vi "SysDef.Import.vi"(8 "error in (no error)":errorcluster, 11 "Path in":path) -> (0 "error out":errorcluster, 3 "Configuration":T1 {"DID Outputs"."Frames"."Signals"."Byte Order" items=["Little Endian", "Big Endian"]; "DID Outputs"."Frames"."Signals"."Data Type" items=["Signed", "Unsigned", "IEEE Float"]; "Memory Inputs"."Frames"."Signals"."Byte Order" items=["Little Endian", "Big Endian"]; "Memory Inputs"."Frames"."Signals"."Data Type" items=["Signed", "Unsigned", "IEEE Float"]; "Memory Outputs"."Frames"."Signals"."Byte Order" items=["Little Endian", "Big Endian"]; "Memory Outputs"."Frames"."Signals"."Data Type" items=["Signed", "Unsigned", "IEEE Float"]; "Routines"."Routine Array"."Stop Parameters"."Response"."Byte Order" items=["Little Endian", "Big Endian"]; "Routines"."Routine Array"."Stop Parameters"."Response"."Data Type" items=["Signed", "Unsigned", "IEEE Float"]; "Routines"."Routine Array"."Stop Parameters"."Cmd"."Byte Order" items=["Little Endian", "Big Endian"]; "Routines"."Routine Array"."Stop Parameters"."Cmd"."Data Type" items=["Signed", "Unsigned", "IEEE Float"]; "Routines"."Routine Array"."Request Parameters"."Response"."Byte Order" items=["Little Endian", "Big Endian"]; "Routines"."Routine Array"."Request Parameters"."Response"."Data Type" items=["Signed", "Unsigned", "IEEE Float"]; "Routines"."Routine Array"."Request Parameters"."Cmd"."Byte Order" items=["Little Endian", "Big Endian"]; "Routines"."Routine Array"."Request Parameters"."Cmd"."Data Type" items=["Signed", "Unsigned", "IEEE Float"]; "Routines"."Routine Array"."Start Parameters"."Response"."Byte Order" items=["Little Endian", "Big Endian"]; "Routines"."Routine Array"."Start Parameters"."Response"."Data Type" items=["Signed", "Unsigned", "IEEE Float"]; "Routines"."Routine Array"."Start Parameters"."Cmd"."Byte Order" items=["Little Endian", "Big Endian"]; "Routines"."Routine Array"."Start Parameters"."Cmd"."Data Type" items=["Signed", "Unsigned", "IEEE Float"]; "IO Controls"."IO Control Array"."Signals"."Response"."Byte Order" items=["Little Endian", "Big Endian"]; "IO Controls"."IO Control Array"."Signals"."Response"."Data Type" items=["Signed", "Unsigned", "IEEE Float"]; "IO Controls"."IO Control Array"."Signals"."Cmd"."Byte Order" items=["Little Endian", "Big Endian"]; "IO Controls"."IO Control Array"."Signals"."Cmd"."Data Type" items=["Signed", "Unsigned", "IEEE Float"]; "DTC"."DTC Control"."Signals"."Byte Order" items=["Little Endian", "Big Endian"]; "DTC"."DTC Control"."Signals"."Data Type" items=["Signed", "Unsigned", "IEEE Float"]; "Diagnostics Basic Configuraiton"."Fill Byte" format="%.0x"; "Diagnostics Basic Configuraiton"."VW TP Channel ID" format="%.0x"; "Diagnostics Basic Configuraiton"."Receive UUDT ID" format="%.0x"; "Diagnostics Basic Configuraiton"."Receive Extension" format="%.0x"; "Diagnostics Basic Configuraiton"."Transmit Extension" format="%.0x"; "Diagnostics Basic Configuraiton"."Receive ID" format="%.0x"; "Diagnostics Basic Configuraiton"."Transmit ID" format="%.0x"; "DID Inputs"."Frames"."Signals"."Byte Order" items=["Little Endian", "Big Endian"]; "DID Inputs"."Frames"."Signals"."Data Type" items=["Signed", "Unsigned", "IEEE Float"]; "PID Inputs"."Frames"."Signals"."Byte Order" items=["Little Endian", "Big Endian"]; "PID Inputs"."Frames"."Signals"."Data Type" items=["Signed", "Unsigned", "IEEE Float"]; "PID Outputs"."Frames"."Signals"."Byte Order" items=["Little Endian", "Big Endian"]; "PID Outputs"."Frames"."Signals"."Data Type" items=["Signed", "Unsigned", "IEEE Float"]})   [LabVIEW 2015, in "Diagnostics Addon System Explorer.lvlib"]
uses:
  Diagnostics Addon System Explorer.lvlib
  Types/SysDef.Export.ctl
  Shared/Types/CAN.ctl
  Shared/Types/CAN.Interface.ctl
  Shared/Types/Protocol.ctl
  Shared/Types/Transport.ctl
  Shared/Types/Security.ctl
  Types/Frames.Export.ctl
  Types/Frame.Export.ctl
  Shared/Types/Signal.ctl
  Types/DPIDs.Export.ctl
  Types/DPID.Export.ctl
  Shared/Types/DPID.ctl
  Shared/Types/DPID.Rate.ctl
  Types/DTC.Export.ctl
  Shared/Types/DTCDescriptor.ctl
  Types/DTCControl.Export.ctl
  Shared/Types/986x.ctl
  Types/Command.Export.ctl
  Types/Status.Export.ctl
  Types/IOControls.Export.ctl
  Types/IO.Export.ctl
  Types/CmdResp.Export.ctl
  Types/Routines.Export.ctl
  Types/Routine.Export.ctl
  Types/UserDefined.Export.ctl
  Types/UserDefined.Group.Export.ctl
  Types/UserDefined.Group.Message.Export.ctl
  <vilib>/NI/GXML/_subVIs/GXML SearchParser/Search Parser.vi
  <vilib>/NI/GXML/GXML.lvlib
  Shared/Diagnostics Addon Shared.lvlib
types:
  T1 = typedef "Diagnostics Addon System Explorer.lvlib/SysDef.Export.ctl" = cluster{"Name":string, "Description":string, "Diagnostics Basic Configuraiton":T2, "DID Outputs":T7, "DID Inputs":T7, "PID Outputs":T7, "PID Inputs":T7, "DPIDs":T10, "DTC":T14, "NI 986x Support":T17, "Commands":T18, "Status":T19, "IO Controls":T20, "Routines":T23, "Memory Outputs":T7, "Memory Inputs":T7, "User Defined":T25}
  T2 = typedef "Diagnostics Addon Shared.lvlib/CAN.ctl" = cluster{"CAN Interface":T3, "Baud Rate":u32, "Diagnostic Protocol":T4, "Transport Protocol":T5, "Transmit ID":u32, "Receive ID":u32, "Transmit Extension":u8, "Receive Extension":u8, "Receive UUDT ID":u32, "Enable Stream":bool, "VW TP Channel ID":u32, "Security":T6, "Fill Frame":bool, "Fill Byte":u8, "Termination":bool}
  T3 = typedef "Diagnostics Addon Shared.lvlib/CAN.Interface.ctl" = string
  T4 = typedef "Diagnostics Addon Shared.lvlib/Protocol.ctl" = enum16{"GMLAN", "KWP-2000", "UDS", "User-Defined"}
  T5 = typedef "Diagnostics Addon Shared.lvlib/Transport.ctl" = enum16{"ISO TP - Normal Mode", "ISO TP - Mixed Mode", "VW TP 2.0", "Diagnostics on IP"}
  T6 = typedef "Diagnostics Addon Shared.lvlib/Security.ctl" = cluster{"Source DLL Path":path, "Security Level":u8, "Target DLL Path":path}
  T7 = typedef "Diagnostics Addon System Explorer.lvlib/Frames.Export.ctl" = cluster{"Description":string, "Frames":T8[]}
  T8 = typedef "Diagnostics Addon System Explorer.lvlib/Frame.Export.ctl" = cluster{"Name":string, "Description":string, "ID":u32, "Signals":T9[]}
  T9 = typedef "Diagnostics Addon Shared.lvlib/Signal.ctl" = cluster{"Start Bit":u32, "Length":u32, "Scaling Factor":dbl, "Scaling Offset":dbl, "Minimum":dbl, "Maximum":dbl, "Data Type":u32, "Byte Order":u32, "Default Value":dbl, "Name":string, "Units":string, "Description":string}
  T10 = typedef "Diagnostics Addon System Explorer.lvlib/DPIDs.Export.ctl" = cluster{"Description":string, "DPIDs":T11[]}
  T11 = typedef "Diagnostics Addon System Explorer.lvlib/DPID.Export.ctl" = cluster{"Name":string, "Description":string, "DPID":T12}
  T12 = typedef "Diagnostics Addon Shared.lvlib/DPID.ctl" = cluster{"DPID ID":u8, "Speed":T13, "PIDs":u16[]}
  T13 = typedef "Diagnostics Addon Shared.lvlib/DPID.Rate.ctl" = enum16{"Slow", "Medium", "Fast"}
  T14 = typedef "Diagnostics Addon System Explorer.lvlib/DTC.Export.ctl" = cluster{"Description":string, "DTC descriptor":T15, "DTC Control":T16, "Created DTCs":u32}
  T15 = typedef "Diagnostics Addon Shared.lvlib/DTCDescriptor.ctl" = cluster{"DTC Byte Length":i32, "Status Byte Length":i32, "Add Data Byte Length":i32, "Byte Order":enum16{"Motorola", "Intel"}}
  T16 = typedef "Diagnostics Addon System Explorer.lvlib/DTCControl.Export.ctl" = cluster{"Description":string, "Signals":T9[]}
  T17 = typedef "Diagnostics Addon Shared.lvlib/986x.ctl" = cluster{"Enable":bool, "RIO Device":string, "Bitfile":path}
  T18 = typedef "Diagnostics Addon System Explorer.lvlib/Command.Export.ctl" = cluster{"Description":string}
  T19 = typedef "Diagnostics Addon System Explorer.lvlib/Status.Export.ctl" = cluster{"Description":string}
  T20 = typedef "Diagnostics Addon System Explorer.lvlib/IOControls.Export.ctl" = cluster{"Description":string, "IO Control Array":T21[]}
  T21 = typedef "Diagnostics Addon System Explorer.lvlib/IO.Export.ctl" = cluster{"Name":string, "Description":string, "ID":u16, "Signals":T22}
  T22 = typedef "Diagnostics Addon System Explorer.lvlib/CmdResp.Export.ctl" = cluster{"Cmd":T9[], "Response":T9[]}
  T23 = typedef "Diagnostics Addon System Explorer.lvlib/Routines.Export.ctl" = cluster{"Description":string, "Routine Array":T24[]}
  T24 = typedef "Diagnostics Addon System Explorer.lvlib/Routine.Export.ctl" = cluster{"Name":string, "Description":string, "ID":u16, "Start Parameters":T22, "Request Parameters":T22, "Stop Parameters":T22}
  T25 = typedef "Diagnostics Addon System Explorer.lvlib/UserDefined.Export.ctl" = cluster{"Description":string, "Groups":T26[]}
  T26 = typedef "Diagnostics Addon System Explorer.lvlib/UserDefined.Group.Export.ctl" = cluster{"Name":string, "Description":string, "Messages":T27[]}
  T27 = typedef "Diagnostics Addon System Explorer.lvlib/UserDefined.Group.Message.Export.ctl" = cluster{"Name":string, "Description":string, "Signals":T22}
  T28 = cluster{"Name":string, "Description":string, "Diagnostics Basic Configuraiton":cluster{"Database File":path, "CAN Interface":enum16{"CAN0", "CAN1", "CAN2", "CAN3", "CAN4", "CAN5", "CAN6", "CAN7", "CAN8", "CAN9", "CAN10", "CAN11", "CAN12", "CAN13", "CAN14", "CAN15", "CAN16", "CAN17", "CAN18", "CAN19", "CAN20", "CAN21", "CAN22", "CAN23", "CAN24", "CAN25", "CAN26", "CAN27", "CAN28", "CAN29", "CAN30", "CAN31", "CAN32", "CAN33", "CAN34", "CAN35", "CAN36", "CAN37", "CAN38", "CAN39", "CAN40", "CAN41", "CAN42", "CAN43", "CAN44", "CAN45", "CAN46", "CAN47", "CAN48", "CAN49", "CAN50", "CAN51", "CAN52", "CAN53", "CAN54", "CAN55", "CAN56", "CAN57", "CAN58", "CAN59", "CAN60", "CAN61", "CAN62", "CAN63", "CAN 256 (Virtual)", "CAN 257 (Virtual)"}, "Baud Rate":u32, "Diagnostic Protocol":enum16{"GMLAN", "KWP-2000", "UDS"}, "Transport Protocol":enum16{"ISO TP - Normal Mode", "ISO TP - Mixed Mode", "VW TP 2.0", "Diagnostics on IP"}, "Transmit ID":u32, "Receive ID":u32, "Transmit Extension":u8, "Receive Extension":u8, "Receive UUDT ID":u32, "Enable Stream":bool, "VW TP Channel ID":u32}, "DIDs":cluster{"Description":string, "DIDPID Array":cluster{"Name":string, "Description":string, "ID":u16, "Signals":cluster{"Name":string, "Start Bit":u8, "Length":u8, "Scaling Factor":dbl, "Scaling Offset":dbl, "Minimum":dbl, "Maximum":dbl, "Data Type":u32, "Byte Order":u32, "Default Value":dbl, "Units":string, "Description":string}[]}[]}, "Input PIDs":cluster{"Description":string, "DIDPID Array":cluster{"Name":string, "Description":string, "ID":u16, "Signals":cluster{"Name":string, "Start Bit":u8, "Length":u8, "Scaling Factor":dbl, "Scaling Offset":dbl, "Minimum":dbl, "Maximum":dbl, "Data Type":u32, "Byte Order":u32, "Default Value":dbl, "Units":string, "Description":string}[]}[]}, "Output PIDs":cluster{"Description":string, "DIDPID Array":cluster{"Name":string, "Description":string, "ID":u16, "Signals":cluster{"Name":string, "Start Bit":u8, "Length":u8, "Scaling Factor":dbl, "Scaling Offset":dbl, "Minimum":dbl, "Maximum":dbl, "Data Type":u32, "Byte Order":u32, "Default Value":dbl, "Units":string, "Description":string}[]}[]}, "DPIDs":cluster{"Description":string, "DPIDs":cluster{"Name":string, "Description":string, "DPID":cluster{"DPID ID":u8, "Speed":enum16{"Slow", "Medium", "Fast"}, "PIDs":u16[]}}[]}, "DTC":cluster{"Description":string, "DTC descriptor":cluster{"DTC Byte Length":i32, "Status Byte Length":i32, "Add Data Byte Length":i32, "Byte Order":enum16{"Motorola", "Intel"}}}, "NI 986x Support":cluster{"Enable 986x":bool, "RIO Device":u16, "Bitfile":path}, "Commands":cluster{"Description":string}, "Status":cluster{"Description":string}}
  T29 = cluster{"Description":string, "DPIDs":cluster{"Name":string, "Description":string, "DPID":cluster{"DPID ID":u8, "Speed":enum16{"Slow", "Medium", "Fast"}, "PIDs":u16[]}}[]}
  T30 = cluster{"DTC Byte Length":i32, "Status Byte Length":i32, "Add Data Byte Length":i32, "Byte Order":enum16{"Motorola", "Intel"}}
  T31 = enum16{"CAN0", "CAN1", "CAN2", "CAN3", "CAN4", "CAN5", "CAN6", "CAN7", "CAN8", "CAN9", "CAN10", "CAN11", "CAN12", "CAN13", "CAN14", "CAN15", "CAN16", "CAN17", "CAN18", "CAN19", "CAN20", "CAN21", "CAN22", "CAN23", "CAN24", "CAN25", "CAN26", "CAN27", "CAN28", "CAN29", "CAN30", "CAN31", "CAN32", "CAN33", "CAN34", "CAN35", "CAN36", "CAN37", "CAN38", "CAN39", "CAN40", "CAN41", "CAN42", "CAN43", "CAN44", "CAN45", "CAN46", "CAN47", "CAN48", "CAN49", "CAN50", "CAN51", "CAN52", "CAN53", "CAN54", "CAN55", "CAN56", "CAN57", "CAN58", "CAN59", "CAN60", "CAN61", "CAN62", "CAN63", "CAN 256 (Virtual)", "CAN 257 (Virtual)"}
  T32 = enum16{"ISO TP - Normal Mode", "ISO TP - Mixed Mode", "VW TP 2.0", "Diagnostics on IP"}
  T33 = cluster{"Name":string, "Description":string, "ID":u16, "Signals":cluster{"Name":string, "Start Bit":u8, "Length":u8, "Scaling Factor":dbl, "Scaling Offset":dbl, "Minimum":dbl, "Maximum":dbl, "Data Type":u32, "Byte Order":u32, "Default Value":dbl, "Units":string, "Description":string}[]}[]
  T34 = cluster{"Name":string, "Description":string, "Diagnostics Basic Configuraiton":cluster{"Database File":path, "CAN Interface":enum16{"CAN0", "CAN1", "CAN2", "CAN3", "CAN4", "CAN5", "CAN6", "CAN7", "CAN8", "CAN9", "CAN10", "CAN11", "CAN12", "CAN13", "CAN14", "CAN15", "CAN16", "CAN17", "CAN18", "CAN19", "CAN20", "CAN21", "CAN22", "CAN23", "CAN24", "CAN25", "CAN26", "CAN27", "CAN28", "CAN29", "CAN30", "CAN31", "CAN32", "CAN33", "CAN34", "CAN35", "CAN36", "CAN37", "CAN38", "CAN39", "CAN40", "CAN41", "CAN42", "CAN43", "CAN44", "CAN45", "CAN46", "CAN47", "CAN48", "CAN49", "CAN50", "CAN51", "CAN52", "CAN53", "CAN54", "CAN55", "CAN56", "CAN57", "CAN58", "CAN59", "CAN60", "CAN61", "CAN62", "CAN63", "CAN 256 (Virtual)", "CAN 257 (Virtual)"}, "Baud Rate":u32, "Diagnostic Protocol":enum16{"GMLAN", "KWP-2000", "UDS"}, "Transport Protocol":enum16{"ISO TP - Normal Mode", "ISO TP - Mixed Mode", "VW TP 2.0", "Diagnostics on IP"}, "Transmit ID":u32, "Receive ID":u32, "Transmit Extension":u8, "Receive Extension":u8, "Receive UUDT ID":u32, "Enable Stream":bool, "VW TP Channel ID":u32}, "DIDs":cluster{"Description":string, "DIDPID Array":cluster{"Name":string, "Description":string, "ID":u16, "Signals":cluster{"Start Bit":u8, "Length":u8, "Scaling Factor":dbl, "Scaling Offset":dbl, "Minimum":dbl, "Maximum":dbl, "Data Type":u32, "Byte Order":u32, "Default Value":dbl, "Name":string, "Units":string, "Description":string}[]}[]}, "Input PIDs":cluster{"Description":string, "DIDPID Array":cluster{"Name":string, "Description":string, "ID":u16, "Signals":cluster{"Start Bit":u8, "Length":u8, "Scaling Factor":dbl, "Scaling Offset":dbl, "Minimum":dbl, "Maximum":dbl, "Data Type":u32, "Byte Order":u32, "Default Value":dbl, "Name":string, "Units":string, "Description":string}[]}[]}, "Output PIDs":cluster{"Description":string, "DIDPID Array":cluster{"Name":string, "Description":string, "ID":u16, "Signals":cluster{"Start Bit":u8, "Length":u8, "Scaling Factor":dbl, "Scaling Offset":dbl, "Minimum":dbl, "Maximum":dbl, "Data Type":u32, "Byte Order":u32, "Default Value":dbl, "Name":string, "Units":string, "Description":string}[]}[]}, "DPIDs":cluster{"Description":string, "DPIDs":cluster{"Name":string, "Description":string, "DPID":cluster{"DPID ID":u8, "Speed":enum16{"Slow", "Medium", "Fast"}, "PIDs":u16[]}}[]}, "DTC":cluster{"Description":string, "DTC descriptor":cluster{"DTC Byte Length":i32, "Status Byte Length":i32, "Add Data Byte Length":i32, "Byte Order":enum16{"Motorola", "Intel"}}}, "NI 986x Support":cluster{"Enable 986x":bool, "RIO Device":u16, "Bitfile":path}, "Commands":cluster{"Description":string}, "Status":cluster{"Description":string}}
  T35 = cluster{"Name":string, "Description":string, "ID":u16, "Signals":cluster{"Start Bit":u8, "Length":u8, "Scaling Factor":dbl, "Scaling Offset":dbl, "Minimum":dbl, "Maximum":dbl, "Data Type":u32, "Byte Order":u32, "Default Value":dbl, "Name":string, "Units":string, "Description":string}[]}[]
  T36 = cluster{"Name":string, "Description":string, "Diagnostics Basic Configuraiton":cluster{"CAN Interface":enum16{"CAN0", "CAN1", "CAN2", "CAN3", "CAN4", "CAN5", "CAN6", "CAN7", "CAN8", "CAN9", "CAN10", "CAN11", "CAN12", "CAN13", "CAN14", "CAN15", "CAN16", "CAN17", "CAN18", "CAN19", "CAN20", "CAN21", "CAN22", "CAN23", "CAN24", "CAN25", "CAN26", "CAN27", "CAN28", "CAN29", "CAN30", "CAN31", "CAN32", "CAN33", "CAN34", "CAN35", "CAN36", "CAN37", "CAN38", "CAN39", "CAN40", "CAN41", "CAN42", "CAN43", "CAN44", "CAN45", "CAN46", "CAN47", "CAN48", "CAN49", "CAN50", "CAN51", "CAN52", "CAN53", "CAN54", "CAN55", "CAN56", "CAN57", "CAN58", "CAN59", "CAN60", "CAN61", "CAN62", "CAN63", "CAN 256 (Virtual)", "CAN 257 (Virtual)"}, "Baud Rate":u32, "Diagnostic Protocol":enum16{"GMLAN", "KWP-2000", "UDS"}, "Transport Protocol":enum16{"ISO TP - Normal Mode", "ISO TP - Mixed Mode", "VW TP 2.0", "Diagnostics on IP"}, "Transmit ID":u32, "Receive ID":u32, "Transmit Extension":u8, "Receive Extension":u8, "Receive UUDT ID":u32, "Enable Stream":bool, "VW TP Channel ID":u32, "Security":cluster{"Source DLL Path":path, "Security Level":u8, "Target DLL Path":path}, "Fill Frame":bool, "Fill Byte":u8, "Termination":bool}, "DID Outputs":cluster{"Description":string, "Frames":cluster{"Name":string, "Description":string, "ID":u32, "Signals":cluster{"Start Bit":u8, "Length":u8, "Scaling Factor":dbl, "Scaling Offset":dbl, "Minimum":dbl, "Maximum":dbl, "Data Type":u32, "Byte Order":u32, "Default Value":dbl, "Name":string, "Units":string, "Description":string}[]}[]}, "DID Inputs":cluster{"Description":string, "Frames":cluster{"Name":string, "Description":string, "ID":u32, "Signals":cluster{"Start Bit":u8, "Length":u8, "Scaling Factor":dbl, "Scaling Offset":dbl, "Minimum":dbl, "Maximum":dbl, "Data Type":u32, "Byte Order":u32, "Default Value":dbl, "Name":string, "Units":string, "Description":string}[]}[]}, "PID Outputs":cluster{"Description":string, "Frames":cluster{"Name":string, "Description":string, "ID":u32, "Signals":cluster{"Start Bit":u8, "Length":u8, "Scaling Factor":dbl, "Scaling Offset":dbl, "Minimum":dbl, "Maximum":dbl, "Data Type":u32, "Byte Order":u32, "Default Value":dbl, "Name":string, "Units":string, "Description":string}[]}[]}, "PID Inputs":cluster{"Description":string, "Frames":cluster{"Name":string, "Description":string, "ID":u32, "Signals":cluster{"Start Bit":u8, "Length":u8, "Scaling Factor":dbl, "Scaling Offset":dbl, "Minimum":dbl, "Maximum":dbl, "Data Type":u32, "Byte Order":u32, "Default Value":dbl, "Name":string, "Units":string, "Description":string}[]}[]}, "DPIDs":cluster{"Description":string, "DPIDs":cluster{"Name":string, "Description":string, "DPID":cluster{"DPID ID":u8, "Speed":enum16{"Slow", "Medium", "Fast"}, "PIDs":u16[]}}[]}, "DTC":cluster{"Description":string, "DTC descriptor":cluster{"DTC Byte Length":i32, "Status Byte Length":i32, "Add Data Byte Length":i32, "Byte Order":enum16{"Motorola", "Intel"}}, "DTC Control":cluster{"Description":string, "Signals":cluster{"Start Bit":u8, "Length":u8, "Scaling Factor":dbl, "Scaling Offset":dbl, "Minimum":dbl, "Maximum":dbl, "Data Type":u32, "Byte Order":u32, "Default Value":dbl, "Name":string, "Units":string, "Description":string}[]}}, "NI 986x Support":cluster{"Enable":bool, "RIO Device":u16, "Bitfile":path}, "Commands":cluster{"Description":string}, "Status":cluster{"Description":string}, "IO Controls":cluster{"Description":string, "IO Control Array":cluster{"Name":string, "Description":string, "ID":u16, "Signals":cluster{"Cmd":cluster{"Start Bit":u8, "Length":u8, "Scaling Factor":dbl, "Scaling Offset":dbl, "Minimum":dbl, "Maximum":dbl, "Data Type":u32, "Byte Order":u32, "Default Value":dbl, "Name":string, "Units":string, "Description":string}[], "Response":cluster{"Start Bit":u8, "Length":u8, "Scaling Factor":dbl, "Scaling Offset":dbl, "Minimum":dbl, "Maximum":dbl, "Data Type":u32, "Byte Order":u32, "Default Value":dbl, "Name":string, "Units":string, "Description":string}[]}}[]}, "Routines":cluster{"Description":string, "Routine Array":cluster{"Name":string, "Description":string, "ID":u16, "Start Parameters":cluster{"Cmd":cluster{"Start Bit":u8, "Length":u8, "Scaling Factor":dbl, "Scaling Offset":dbl, "Minimum":dbl, "Maximum":dbl, "Data Type":u32, "Byte Order":u32, "Default Value":dbl, "Name":string, "Units":string, "Description":string}[], "Response":cluster{"Start Bit":u8, "Length":u8, "Scaling Factor":dbl, "Scaling Offset":dbl, "Minimum":dbl, "Maximum":dbl, "Data Type":u32, "Byte Order":u32, "Default Value":dbl, "Name":string, "Units":string, "Description":string}[]}, "Request Parameters":cluster{"Cmd":cluster{"Start Bit":u8, "Length":u8, "Scaling Factor":dbl, "Scaling Offset":dbl, "Minimum":dbl, "Maximum":dbl, "Data Type":u32, "Byte Order":u32, "Default Value":dbl, "Name":string, "Units":string, "Description":string}[], "Response":cluster{"Start Bit":u8, "Length":u8, "Scaling Factor":dbl, "Scaling Offset":dbl, "Minimum":dbl, "Maximum":dbl, "Data Type":u32, "Byte Order":u32, "Default Value":dbl, "Name":string, "Units":string, "Description":string}[]}, "Stop Parameters":cluster{"Cmd":cluster{"Start Bit":u8, "Length":u8, "Scaling Factor":dbl, "Scaling Offset":dbl, "Minimum":dbl, "Maximum":dbl, "Data Type":u32, "Byte Order":u32, "Default Value":dbl, "Name":string, "Units":string, "Description":string}[], "Response":cluster{"Start Bit":u8, "Length":u8, "Scaling Factor":dbl, "Scaling Offset":dbl, "Minimum":dbl, "Maximum":dbl, "Data Type":u32, "Byte Order":u32, "Default Value":dbl, "Name":string, "Units":string, "Description":string}[]}}[]}, "Memory Outputs":cluster{"Description":string, "Frames":cluster{"Name":string, "Description":string, "ID":u32, "Signals":cluster{"Start Bit":u8, "Length":u8, "Scaling Factor":dbl, "Scaling Offset":dbl, "Minimum":dbl, "Maximum":dbl, "Data Type":u32, "Byte Order":u32, "Default Value":dbl, "Name":string, "Units":string, "Description":string}[]}[]}, "Memory Inputs":cluster{"Description":string, "Frames":cluster{"Name":string, "Description":string, "ID":u32, "Signals":cluster{"Start Bit":u8, "Length":u8, "Scaling Factor":dbl, "Scaling Offset":dbl, "Minimum":dbl, "Maximum":dbl, "Data Type":u32, "Byte Order":u32, "Default Value":dbl, "Name":string, "Units":string, "Description":string}[]}[]}}
  T37 = cluster{"Description":string, "Frames":cluster{"Name":string, "Description":string, "ID":u32, "Signals":cluster{"Start Bit":u8, "Length":u8, "Scaling Factor":dbl, "Scaling Offset":dbl, "Minimum":dbl, "Maximum":dbl, "Data Type":u32, "Byte Order":u32, "Default Value":dbl, "Name":string, "Units":string, "Description":string}[]}[]}
  T38 = cluster{"Description":string, "Signals":cluster{"Start Bit":u8, "Length":u8, "Scaling Factor":dbl, "Scaling Offset":dbl, "Minimum":dbl, "Maximum":dbl, "Data Type":u32, "Byte Order":u32, "Default Value":dbl, "Name":string, "Units":string, "Description":string}[]}
  T39 = cluster{"Description":string, "IO Control Array":cluster{"Name":string, "Description":string, "ID":u16, "Signals":cluster{"Cmd":cluster{"Start Bit":u8, "Length":u8, "Scaling Factor":dbl, "Scaling Offset":dbl, "Minimum":dbl, "Maximum":dbl, "Data Type":u32, "Byte Order":u32, "Default Value":dbl, "Name":string, "Units":string, "Description":string}[], "Response":cluster{"Start Bit":u8, "Length":u8, "Scaling Factor":dbl, "Scaling Offset":dbl, "Minimum":dbl, "Maximum":dbl, "Data Type":u32, "Byte Order":u32, "Default Value":dbl, "Name":string, "Units":string, "Description":string}[]}}[]}
  T40 = cluster{"Description":string, "Routine Array":cluster{"Name":string, "Description":string, "ID":u16, "Start Parameters":cluster{"Cmd":cluster{"Start Bit":u8, "Length":u8, "Scaling Factor":dbl, "Scaling Offset":dbl, "Minimum":dbl, "Maximum":dbl, "Data Type":u32, "Byte Order":u32, "Default Value":dbl, "Name":string, "Units":string, "Description":string}[], "Response":cluster{"Start Bit":u8, "Length":u8, "Scaling Factor":dbl, "Scaling Offset":dbl, "Minimum":dbl, "Maximum":dbl, "Data Type":u32, "Byte Order":u32, "Default Value":dbl, "Name":string, "Units":string, "Description":string}[]}, "Request Parameters":cluster{"Cmd":cluster{"Start Bit":u8, "Length":u8, "Scaling Factor":dbl, "Scaling Offset":dbl, "Minimum":dbl, "Maximum":dbl, "Data Type":u32, "Byte Order":u32, "Default Value":dbl, "Name":string, "Units":string, "Description":string}[], "Response":cluster{"Start Bit":u8, "Length":u8, "Scaling Factor":dbl, "Scaling Offset":dbl, "Minimum":dbl, "Maximum":dbl, "Data Type":u32, "Byte Order":u32, "Default Value":dbl, "Name":string, "Units":string, "Description":string}[]}, "Stop Parameters":cluster{"Cmd":cluster{"Start Bit":u8, "Length":u8, "Scaling Factor":dbl, "Scaling Offset":dbl, "Minimum":dbl, "Maximum":dbl, "Data Type":u32, "Byte Order":u32, "Default Value":dbl, "Name":string, "Units":string, "Description":string}[], "Response":cluster{"Start Bit":u8, "Length":u8, "Scaling Factor":dbl, "Scaling Offset":dbl, "Minimum":dbl, "Maximum":dbl, "Data Type":u32, "Byte Order":u32, "Default Value":dbl, "Name":string, "Units":string, "Description":string}[]}}[]}
  T41 = cluster{"Source DLL Path":path, "Security Level":u8, "Target DLL Path":path}
  T42 = cluster{"Name":string, "Description":string, "Diagnostics Basic Configuraiton":cluster{"CAN Interface":enum16{"CAN0", "CAN1", "CAN2", "CAN3", "CAN4", "CAN5", "CAN6", "CAN7", "CAN8", "CAN9", "CAN10", "CAN11", "CAN12", "CAN13", "CAN14", "CAN15", "CAN16", "CAN17", "CAN18", "CAN19", "CAN20", "CAN21", "CAN22", "CAN23", "CAN24", "CAN25", "CAN26", "CAN27", "CAN28", "CAN29", "CAN30", "CAN31", "CAN32", "CAN33", "CAN34", "CAN35", "CAN36", "CAN37", "CAN38", "CAN39", "CAN40", "CAN41", "CAN42", "CAN43", "CAN44", "CAN45", "CAN46", "CAN47", "CAN48", "CAN49", "CAN50", "CAN51", "CAN52", "CAN53", "CAN54", "CAN55", "CAN56", "CAN57", "CAN58", "CAN59", "CAN60", "CAN61", "CAN62", "CAN63", "CAN 256 (Virtual)", "CAN 257 (Virtual)"}, "Baud Rate":u32, "Diagnostic Protocol":T4, "Transport Protocol":T5, "Transmit ID":u32, "Receive ID":u32, "Transmit Extension":u8, "Receive Extension":u8, "Receive UUDT ID":u32, "Enable Stream":bool, "VW TP Channel ID":u32, "Security":T6, "Fill Frame":bool, "Fill Byte":u8, "Termination":bool}, "DID Outputs":T7, "DID Inputs":T7, "PID Outputs":T7, "PID Inputs":T7, "DPIDs":T10, "DTC":T14, "NI 986x Support":cluster{"Enable":bool, "RIO Device":u16, "Bitfile":path}, "Commands":T18, "Status":T19, "IO Controls":T20, "Routines":T23, "Memory Outputs":T7, "Memory Inputs":T7, "User Defined":T25}
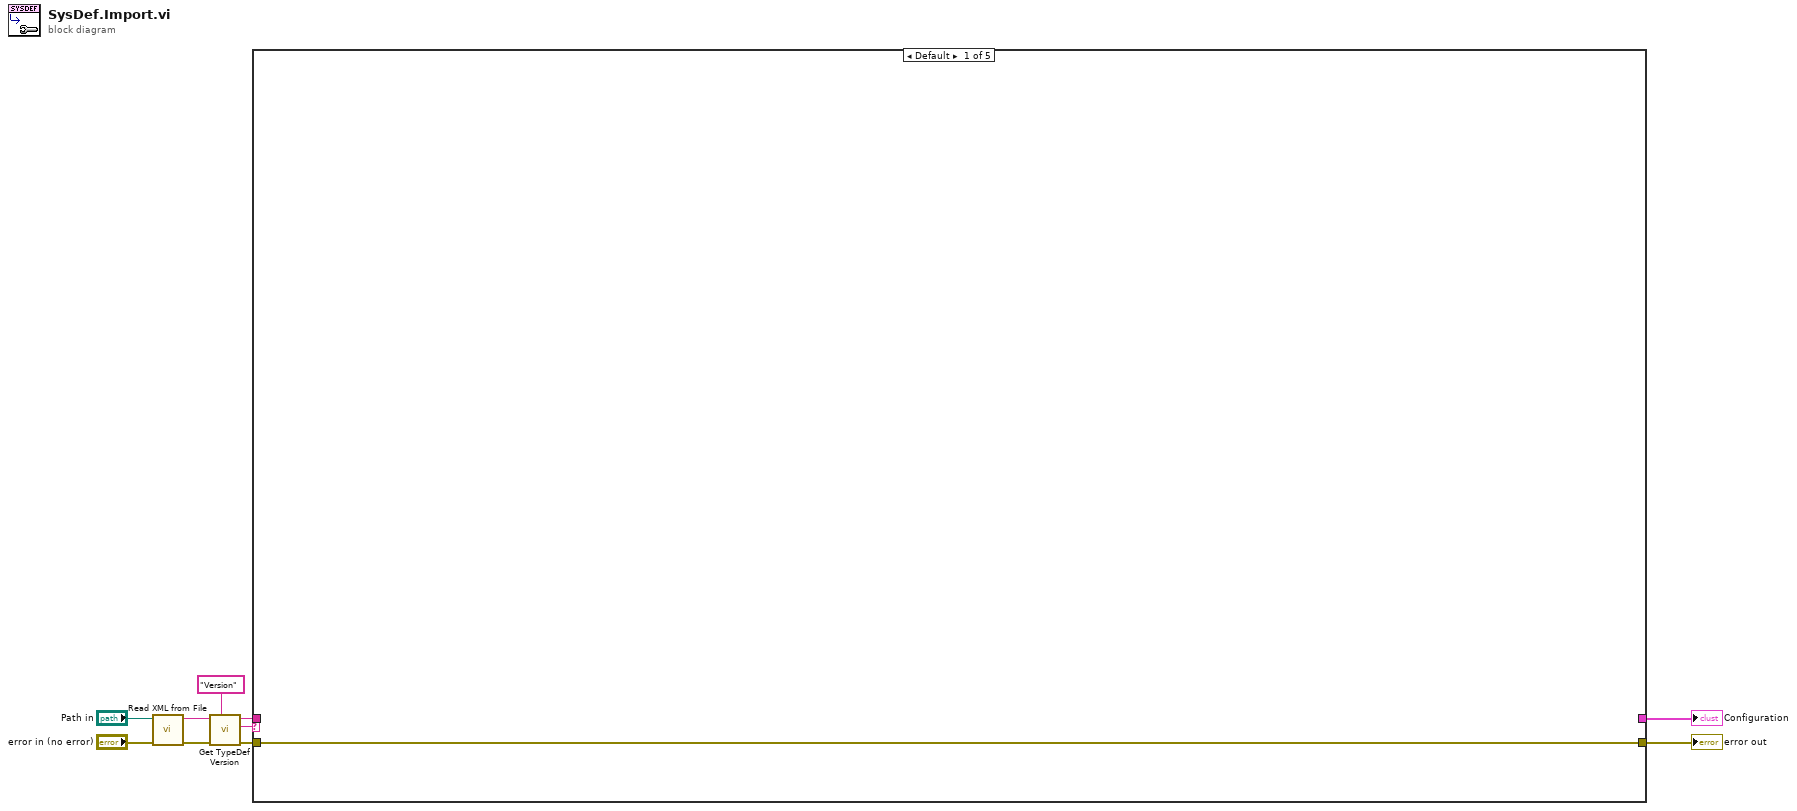
[diagram p0: block diagram]
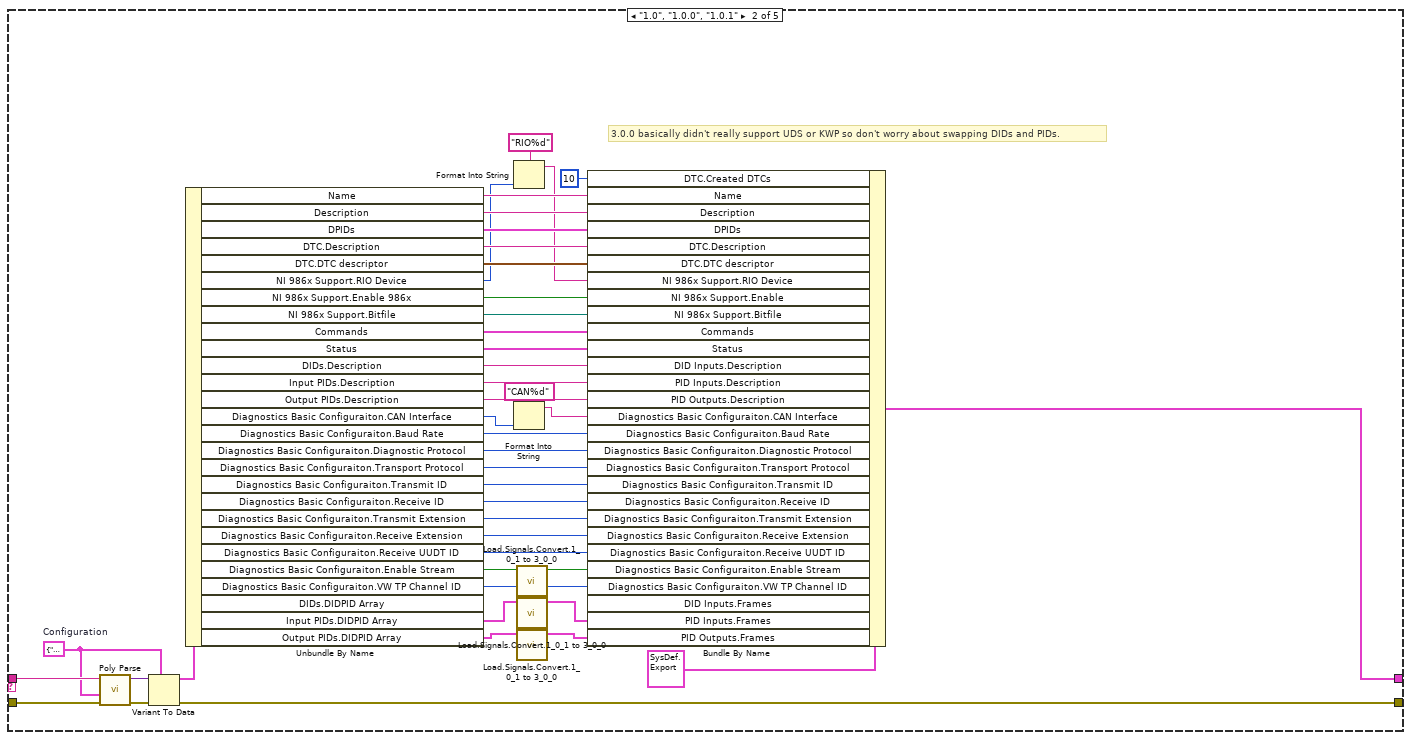
[diagram p2: hidden frame]
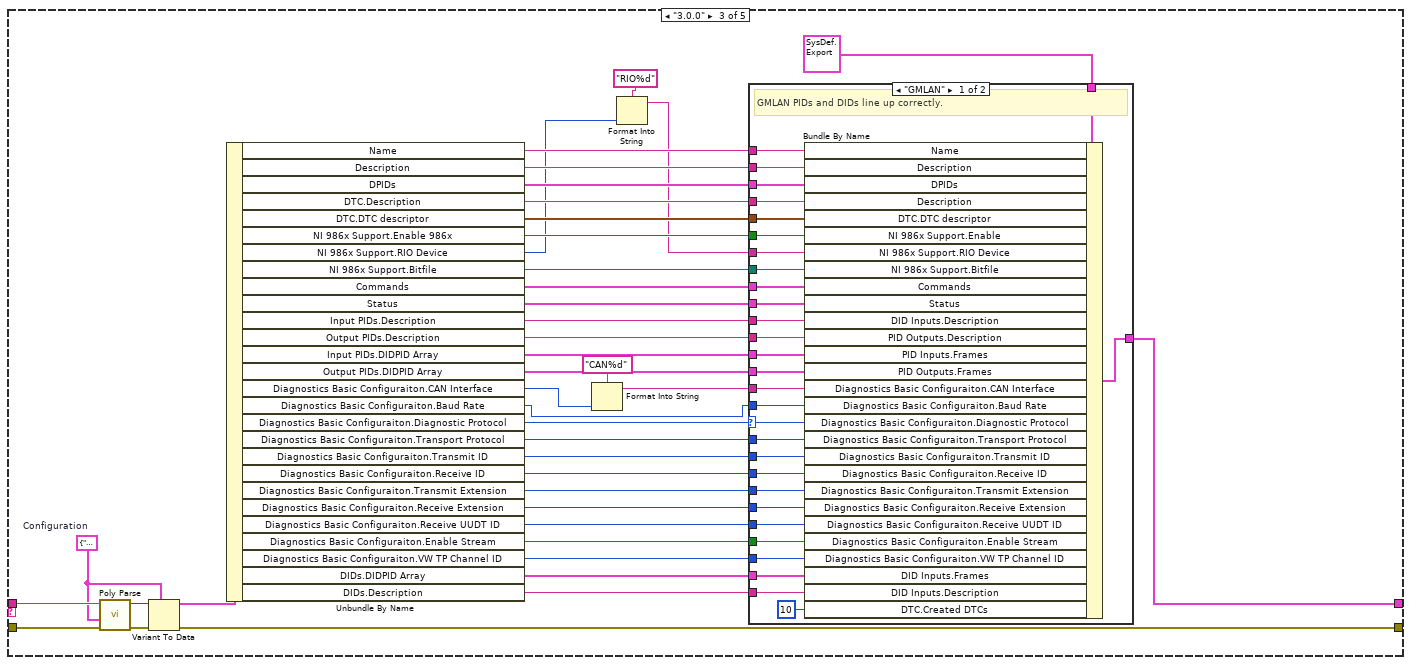
[diagram p3: hidden frame]
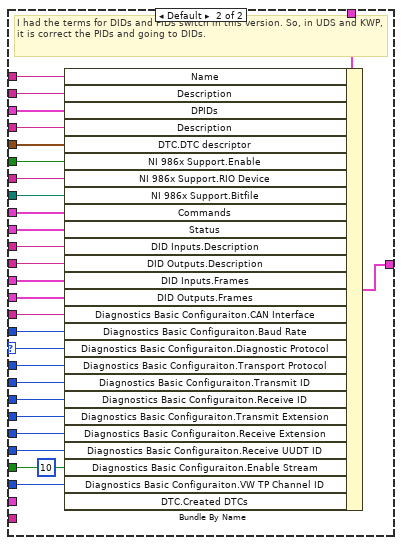
[diagram p4: hidden frame]
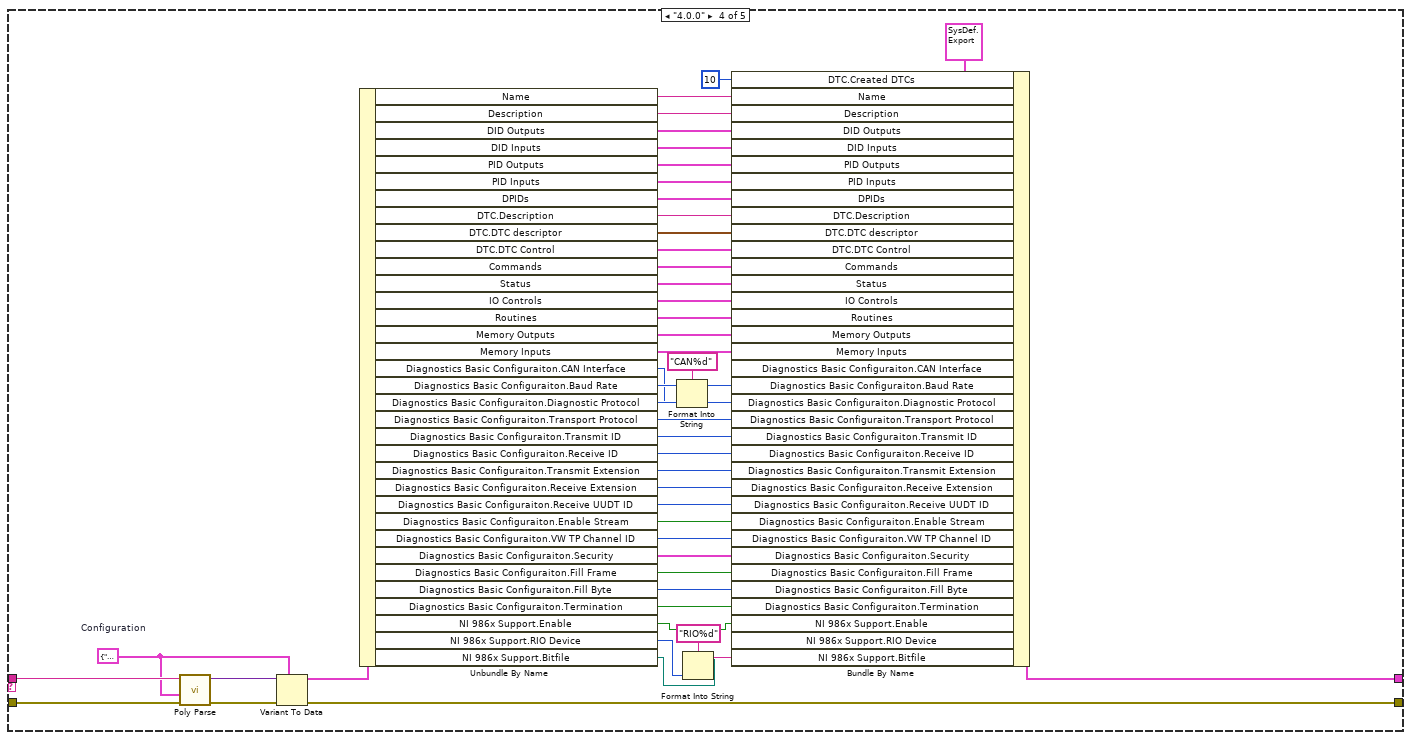
[diagram p5: hidden frame]
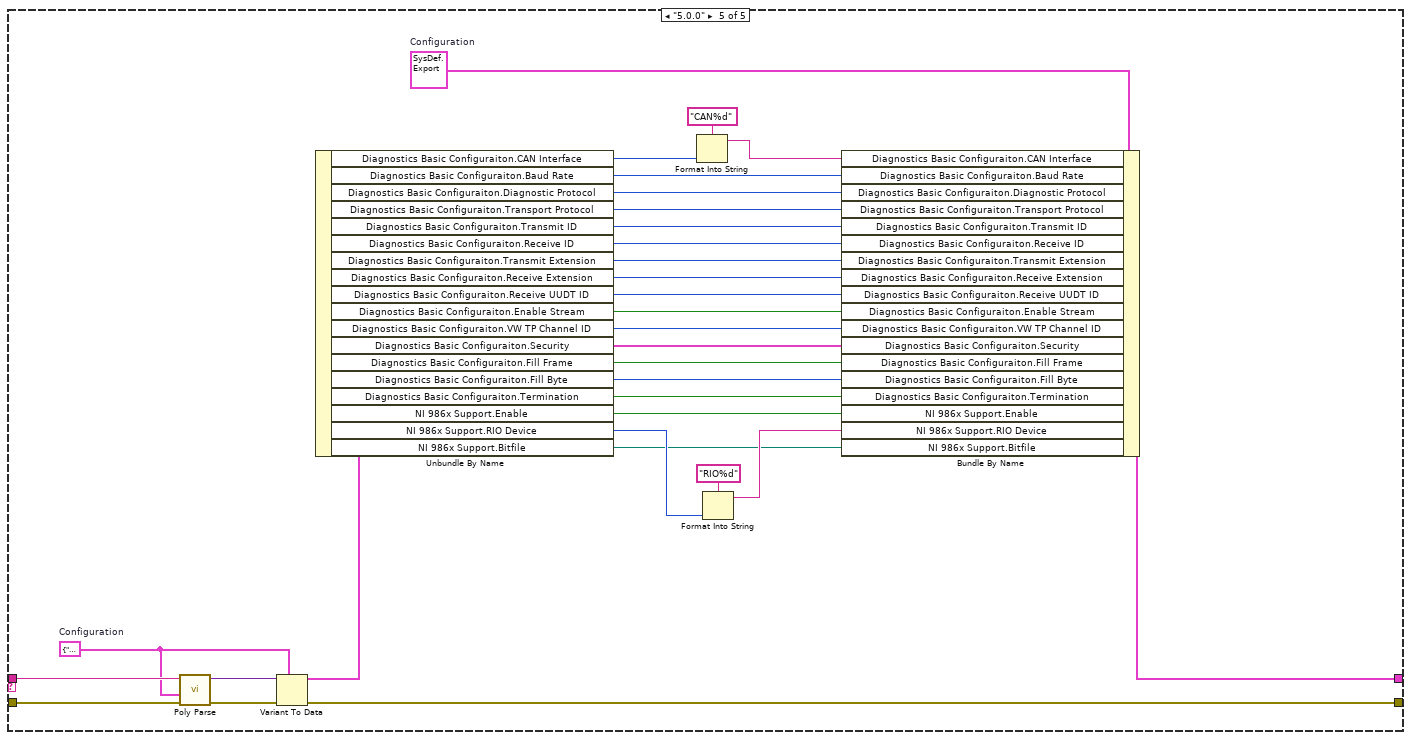
[diagram p6: hidden frame]
diagram:
  n1 = call <vilib>:"Read XML from File.vi"("error in"="error in (no error)", "XML File Path"="Path in") -> ("error out"=w1:errorcluster, "XML String Out"=w2:string)  [unwired: 8 in]
  n2 = call <vilib>:"Get TypeDef Version.vi"("Version Tag Name"="Version", "error in"=w1, "XML String In"=w2) -> ("error out"=w5:errorcluster, "Version String"=w6:string, "XML String Out"=w4:string)  [unwired: 6 in]
  n3 = case shown="Default" w6 {
    tunnel: w4 -> [_ w55 w95 w201 w232]
    tunnel: w5 -> [w11 w54 w94 w200 w231]
    tunnel: [_ w39 w89 w179 w224] -> w10
    tunnel: [w11 w51 w91 w197 w228] -> w9
    frame Default {
    }
    frame "1.0", "1.0.0", "1.0.1" {
      w38 = T28 {"Name"="", "Description"="", "Diagnostics Basic Configuraiton"={"Database File"=path "", "CAN Interface"=enum."CAN0", "Baud Rate"=0, "Diagnostic Protocol"=enum."GMLAN", "Transport Protocol"=enum."ISO TP - Normal Mode", "Transmit ID"=0, "Receive ID"=0, "Transmit Extension"=0, "Receive Extension"=0, "Receive UUDT ID"=0, "Enable Stream"=FALSE, "VW TP Channel ID"=0}, "DIDs"={"Description"="", "DIDPID Array"=[]}, "Input PIDs"={"Description"="", "DIDPID Array"=[]}, "Output PIDs"={"Description"="", "DIDPID Array"=[]}, "DPIDs"={"Description"="", "DPIDs"=[]}, "DTC"={"Description"="", "DTC descriptor"={"DTC Byte Length"=0, "Status Byte Length"=0, "Add Data Byte Length"=0, "Byte Order"=enum."Motorola"}}, "NI 986x Support"={"Enable 986x"=FALSE, "RIO Device"=0, "Bitfile"=path ""}, "Commands"={"Description"=""}, "Status"={"Description"=""}}  # Configuration
      # "3.0.0 basically didn't really support UDS or KWP so don't worry about swapping DIDs and PIDs."
      n4 = call-poly <vilib>:"Poly Parse.vi"("error in"=w54, "TypeDesc"=w38, "XML String In"=w55) -> ("error out"=w53:errorcluster, "Parsed Data"=w52:variant)  [unwired: 7 in]
      n5 = Variant To Data(error in=w53, type=w38, Variant=w52) -> (data=w50:T28, error out=w51:errorcluster)
      n6 = Unbundle By Name(w50) -> ("Name"=w49:string, "Description"=w48:string, "DPIDs"=w47:T29, "DTC.Description"=w43:string, "DTC.DTC descriptor"=w21:T30, "NI 986x Support.RIO Device"=w13:u16, "NI 986x Support.Enable 986x"=w14:bool, "NI 986x Support.Bitfile"=w44:path, "Commands"=w45:cluster{"Description":string}, "Status"=w46:cluster{"Description":string}, "DIDs.Description"=w42:string, "Input PIDs.Description"=w41:string, "Output PIDs.Description"=w40:string, "Diagnostics Basic Configuraiton.CAN Interface"=w18:T31, "Diagnostics Basic Configuraiton.Baud Rate"=w28:u32, "Diagnostics Basic Configuraiton.Diagnostic Protocol"=w29:enum16{"GMLAN", "KWP-2000", "UDS"}, "Diagnostics Basic Configuraiton.Transport Protocol"=w30:T32, "Diagnostics Basic Configuraiton.Transmit ID"=w31:u32, "Diagnostics Basic Configuraiton.Receive ID"=w32:u32, "Diagnostics Basic Configuraiton.Transmit Extension"=w33:u8, "Diagnostics Basic Configuraiton.Receive Extension"=w34:u8, "Diagnostics Basic Configuraiton.Receive UUDT ID"=w35:u32, "Diagnostics Basic Configuraiton.Enable Stream"=w36:bool, "Diagnostics Basic Configuraiton.VW TP Channel ID"=w37:u32, "DIDs.DIDPID Array"=w27:T33, "Input PIDs.DIDPID Array"=w26:T33, "Output PIDs.DIDPID Array"=w25:T33)
      n7 = Format Into String(format string="RIO%d", w13) -> (resulting string=w12:string)  [unwired: 2 in, 1 out]
      n8 = Format Into String(format string="CAN%d", w18) -> (resulting string=w17:string)  [unwired: 2 in, 1 out]
      n9 = call "Load.Signals.Convert.1_0_1 to 3_0_0.vi"("Signals"=w27) -> ("Signals"=w24:T8[])  [unwired: 10 in]
      n10 = call "Load.Signals.Convert.1_0_1 to 3_0_0.vi"("Signals"=w26) -> ("Signals"=w23:T8[])  [unwired: 10 in]
      n11 = call "Load.Signals.Convert.1_0_1 to 3_0_0.vi"("Signals"=w25) -> ("Signals"=w22:T8[])  [unwired: 10 in]
      n12 = Bundle By Name(cluster=T1 {"Name"="", "Description"="", "Diagnostics Basic Configuraiton"={"CAN Interface"="", "Baud Rate"=0, "Diagnostic Protocol"=enum."GMLAN", "Transport Protocol"=enum."ISO TP - Normal Mode", "Transmit ID"=0, "Receive ID"=0, "Transmit Extension"=0, "Receive Extension"=0, "Receive UUDT ID"=0, "Enable Stream"=TRUE, "VW TP Channel ID"=0, "Security"={"Source DLL Path"=path "", "Security Level"=1, "Target DLL Path"=path ""}, "Fill Frame"=FALSE, "Fill Byte"=255, "Termination"=FALSE}, "DID Outputs"={"Description"="", "Frames"=[]}, "DID Inputs"={"Description"="", "Frames"=[]}, "PID Outputs"={"Description"="", "Frames"=[]}, "PID Inputs"={"Description"="", "Frames"=[]}, "DPIDs"={"Description"="", "DPIDs"=[]}, "DTC"={"Description"="", "DTC descriptor"={"DTC Byte Length"=2, "Status Byte Length"=1, "Add Data Byte Length"=1, "Byte Order"=enum."Motorola"}, "DTC Control"={"Description"="", "Signals"=[]}, "Created DTCs"=0}, "NI 986x Support"={"Enable"=FALSE, "RIO Device"="", "Bitfile"=path ""}, "Commands"={"Description"=""}, "Status"={"Description"=""}, "IO Controls"={"Description"="", "IO Control Array"=[]}, "Routines"={"Description"="", "Routine Array"=[]}, "Memory Outputs"={"Description"="", "Frames"=[]}, "Memory Inputs"={"Description"="", "Frames"=[]}, "User Defined"={"Description"="", "Groups"=[]}} ("Configuration"), "DTC.Created DTCs"=u32 10, "Name"=w49, "Description"=w48, "DPIDs"=w47, "DTC.Description"=w43, "DTC.DTC descriptor"=w21, "NI 986x Support.RIO Device"=w12, "NI 986x Support.Enable"=w14, "NI 986x Support.Bitfile"=w44, "Commands"=w45, "Status"=w46, "DID Inputs.Description"=w42, "PID Inputs.Description"=w41, "PID Outputs.Description"=w40, "Diagnostics Basic Configuraiton.CAN Interface"=w17, "Diagnostics Basic Configuraiton.Baud Rate"=w28, "Diagnostics Basic Configuraiton.Diagnostic Protocol"=w29, "Diagnostics Basic Configuraiton.Transport Protocol"=w30, "Diagnostics Basic Configuraiton.Transmit ID"=w31, "Diagnostics Basic Configuraiton.Receive ID"=w32, "Diagnostics Basic Configuraiton.Transmit Extension"=w33, "Diagnostics Basic Configuraiton.Receive Extension"=w34, "Diagnostics Basic Configuraiton.Receive UUDT ID"=w35, "Diagnostics Basic Configuraiton.Enable Stream"=w36, "Diagnostics Basic Configuraiton.VW TP Channel ID"=w37, "DID Inputs.Frames"=w24, "PID Inputs.Frames"=w23, "PID Outputs.Frames"=w22) -> (w39:T1)
    }
    frame "3.0.0" {
      w88 = T34 {"Name"="", "Description"="", "Diagnostics Basic Configuraiton"={"Database File"=path "", "CAN Interface"=enum."CAN0", "Baud Rate"=0, "Diagnostic Protocol"=enum."GMLAN", "Transport Protocol"=enum."ISO TP - Normal Mode", "Transmit ID"=0, "Receive ID"=0, "Transmit Extension"=0, "Receive Extension"=0, "Receive UUDT ID"=0, "Enable Stream"=FALSE, "VW TP Channel ID"=0}, "DIDs"={"Description"="", "DIDPID Array"=[]}, "Input PIDs"={"Description"="", "DIDPID Array"=[]}, "Output PIDs"={"Description"="", "DIDPID Array"=[]}, "DPIDs"={"Description"="", "DPIDs"=[]}, "DTC"={"Description"="", "DTC descriptor"={"DTC Byte Length"=0, "Status Byte Length"=0, "Add Data Byte Length"=0, "Byte Order"=enum."Motorola"}}, "NI 986x Support"={"Enable 986x"=FALSE, "RIO Device"=0, "Bitfile"=path ""}, "Commands"={"Description"=""}, "Status"={"Description"=""}}  # Configuration
      n13 = call-poly <vilib>:"Poly Parse.vi"("error in"=w94, "TypeDesc"=w88, "XML String In"=w95) -> ("error out"=w93:errorcluster, "Parsed Data"=w92:variant)  [unwired: 7 in]
      n14 = Variant To Data(error in=w93, type=w88, Variant=w92) -> (data=w90:T34, error out=w91:errorcluster)
      n15 = Unbundle By Name(w90) -> ("Name"=w87:string, "Description"=w86:string, "DPIDs"=w85:T29, "DTC.Description"=w81:string, "DTC.DTC descriptor"=w67:T30, "NI 986x Support.Enable 986x"=w82:bool, "NI 986x Support.RIO Device"=w57:u16, "NI 986x Support.Bitfile"=w58:path, "Commands"=w83:cluster{"Description":string}, "Status"=w84:cluster{"Description":string}, "Input PIDs.Description"=w80:string, "Output PIDs.Description"=w79:string, "Input PIDs.DIDPID Array"=w78:T35, "Output PIDs.DIDPID Array"=w77:T35, "Diagnostics Basic Configuraiton.CAN Interface"=w61:T31, "Diagnostics Basic Configuraiton.Baud Rate"=w68:u32, "Diagnostics Basic Configuraiton.Diagnostic Protocol"=w65:enum16{"GMLAN", "KWP-2000", "UDS"}, "Diagnostics Basic Configuraiton.Transport Protocol"=w69:T32, "Diagnostics Basic Configuraiton.Transmit ID"=w70:u32, "Diagnostics Basic Configuraiton.Receive ID"=w71:u32, "Diagnostics Basic Configuraiton.Transmit Extension"=w72:u8, "Diagnostics Basic Configuraiton.Receive Extension"=w73:u8, "Diagnostics Basic Configuraiton.Receive UUDT ID"=w74:u32, "Diagnostics Basic Configuraiton.Enable Stream"=w75:bool, "Diagnostics Basic Configuraiton.VW TP Channel ID"=w76:u32, "DIDs.DIDPID Array"=w64:T35, "DIDs.Description"=w63:string)
      n16 = Format Into String(format string="CAN%d", w61) -> (resulting string=w60:string)  [unwired: 2 in, 1 out]
      n17 = Format Into String(format string="RIO%d", w57) -> (resulting string=w56:string)  [unwired: 2 in, 1 out]
      n18 = case shown="\"GMLAN\"" w65 {
        selector: w65 -> [w103 w129]
        tunnel: [w125 w153] -> w89
        tunnel: w87 -> [w124 w152]
        tunnel: w86 -> [w123 w151]
        tunnel: w85 -> [w122 w150]
        tunnel: w84 -> [w121 w149]
        tunnel: w83 -> [w120 w148]
        tunnel: w82 -> [w119 w147]
        tunnel: w81 -> [w118 w146]
        tunnel: w80 -> [w117 w145]
        tunnel: w79 -> [w116 w144]
        tunnel: w78 -> [w99 w143]
        tunnel: w77 -> [w100 w142]
        tunnel: w76 -> [w115 w141]
        tunnel: w75 -> [w114 w140]
        tunnel: w74 -> [w113 w139]
        tunnel: w73 -> [w112 w138]
        tunnel: w72 -> [w111 w137]
        tunnel: w71 -> [w110 w136]
        tunnel: w70 -> [w109 w135]
        tunnel: w69 -> [w108 w134]
        tunnel: w68 -> [w107 w133]
        tunnel: w60 -> [w106 w132]
        tunnel: w67 -> [w105 w131]
        tunnel: T1 {"Name"="", "Description"="", "Diagnostics Basic Configuraiton"={"CAN Interface"="", "Baud Rate"=0, "Diagnostic Protocol"=enum."GMLAN", "Transport Protocol"=enum."ISO TP - Normal Mode", "Transmit ID"=0, "Receive ID"=0, "Transmit Extension"=0, "Receive Extension"=0, "Receive UUDT ID"=0, "Enable Stream"=TRUE, "VW TP Channel ID"=0, "Security"={"Source DLL Path"=path "", "Security Level"=1, "Target DLL Path"=path ""}, "Fill Frame"=FALSE, "Fill Byte"=255, "Termination"=FALSE}, "DID Outputs"={"Description"="", "Frames"=[]}, "DID Inputs"={"Description"="", "Frames"=[]}, "PID Outputs"={"Description"="", "Frames"=[]}, "PID Inputs"={"Description"="", "Frames"=[]}, "DPIDs"={"Description"="", "DPIDs"=[]}, "DTC"={"Description"="", "DTC descriptor"={"DTC Byte Length"=2, "Status Byte Length"=1, "Add Data Byte Length"=1, "Byte Order"=enum."Motorola"}, "DTC Control"={"Description"="", "Signals"=[]}, "Created DTCs"=0}, "NI 986x Support"={"Enable"=FALSE, "RIO Device"="", "Bitfile"=path ""}, "Commands"={"Description"=""}, "Status"={"Description"=""}, "IO Controls"={"Description"="", "IO Control Array"=[]}, "Routines"={"Description"="", "Routine Array"=[]}, "Memory Outputs"={"Description"="", "Frames"=[]}, "Memory Inputs"={"Description"="", "Frames"=[]}, "User Defined"={"Description"="", "Groups"=[]}} ("Configuration") -> [w104 w130]
        tunnel: w64 -> [w102 _]
        tunnel: w63 -> [w101 _]
        tunnel: w58 -> [w97 w127]
        tunnel: w56 -> [w96 w126]
        frame "GMLAN" {
          # "GMLAN PIDs and DIDs line up correctly."
          n19 = Bundle By Name(cluster=w104, "Name"=w124, "Description"=w123, "DPIDs"=w122, "Description"=w118, "DTC.DTC descriptor"=w105, "NI 986x Support.Enable"=w119, "NI 986x Support.RIO Device"=w96, "NI 986x Support.Bitfile"=w97, "Commands"=w120, "Status"=w121, "DID Inputs.Description"=w117, "PID Outputs.Description"=w116, "PID Inputs.Frames"=w99, "PID Outputs.Frames"=w100, "Diagnostics Basic Configuraiton.CAN Interface"=w106, "Diagnostics Basic Configuraiton.Baud Rate"=w107, "Diagnostics Basic Configuraiton.Diagnostic Protocol"=w103, "Diagnostics Basic Configuraiton.Transport Protocol"=w108, "Diagnostics Basic Configuraiton.Transmit ID"=w109, "Diagnostics Basic Configuraiton.Receive ID"=w110, "Diagnostics Basic Configuraiton.Transmit Extension"=w111, "Diagnostics Basic Configuraiton.Receive Extension"=w112, "Diagnostics Basic Configuraiton.Receive UUDT ID"=w113, "Diagnostics Basic Configuraiton.Enable Stream"=w114, "Diagnostics Basic Configuraiton.VW TP Channel ID"=w115, "DID Inputs.Frames"=w102, "DID Inputs.Description"=w101, "DTC.Created DTCs"=u32 10) -> (w125:T1)
        }
        frame Default {
          # "I had the terms for DIDs and PIDs switch in this version. So, in UDS and KWP, it is correct the PIDs and going to DIDs."
          n20 = Bundle By Name(cluster=w130, "Name"=w152, "Description"=w151, "DPIDs"=w150, "Description"=w146, "DTC.DTC descriptor"=w131, "NI 986x Support.Enable"=w147, "NI 986x Support.RIO Device"=w126, "NI 986x Support.Bitfile"=w127, "Commands"=w148, "Status"=w149, "DID Inputs.Description"=w145, "DID Outputs.Description"=w144, "DID Inputs.Frames"=w143, "DID Outputs.Frames"=w142, "Diagnostics Basic Configuraiton.CAN Interface"=w132, "Diagnostics Basic Configuraiton.Baud Rate"=w133, "Diagnostics Basic Configuraiton.Diagnostic Protocol"=w129, "Diagnostics Basic Configuraiton.Transport Protocol"=w134, "Diagnostics Basic Configuraiton.Transmit ID"=w135, "Diagnostics Basic Configuraiton.Receive ID"=w136, "Diagnostics Basic Configuraiton.Transmit Extension"=w137, "Diagnostics Basic Configuraiton.Receive Extension"=w138, "Diagnostics Basic Configuraiton.Receive UUDT ID"=w139, "Diagnostics Basic Configuraiton.Enable Stream"=w140, "Diagnostics Basic Configuraiton.VW TP Channel ID"=w141, "DTC.Created DTCs"=u32 10) -> (w153:T1)
        }
      }
    }
    frame "4.0.0" {
      w196 = T36 {"Name"="", "Description"="", "Diagnostics Basic Configuraiton"={"CAN Interface"=enum."CAN0", "Baud Rate"=0, "Diagnostic Protocol"=enum."GMLAN", "Transport Protocol"=enum."ISO TP - Normal Mode", "Transmit ID"=0, "Receive ID"=0, "Transmit Extension"=0, "Receive Extension"=0, "Receive UUDT ID"=0, "Enable Stream"=TRUE, "VW TP Channel ID"=0, "Security"={"Source DLL Path"=path "", "Security Level"=1, "Target DLL Path"=path ""}, "Fill Frame"=FALSE, "Fill Byte"=255, "Termination"=FALSE}, "DID Outputs"={"Description"="", "Frames"=[]}, "DID Inputs"={"Description"="", "Frames"=[]}, "PID Outputs"={"Description"="", "Frames"=[]}, "PID Inputs"={"Description"="", "Frames"=[]}, "DPIDs"={"Description"="", "DPIDs"=[]}, "DTC"={"Description"="", "DTC descriptor"={"DTC Byte Length"=2, "Status Byte Length"=1, "Add Data Byte Length"=1, "Byte Order"=enum."Motorola"}, "DTC Control"={"Description"="", "Signals"=[]}}, "NI 986x Support"={"Enable"=FALSE, "RIO Device"=0, "Bitfile"=path ""}, "Commands"={"Description"=""}, "Status"={"Description"=""}, "IO Controls"={"Description"="", "IO Control Array"=[]}, "Routines"={"Description"="", "Routine Array"=[]}, "Memory Outputs"={"Description"="", "Frames"=[]}, "Memory Inputs"={"Description"="", "Frames"=[]}}  # Configuration
      n21 = call-poly <vilib>:"Poly Parse.vi"("error in"=w200, "TypeDesc"=w196, "XML String In"=w201) -> ("error out"=w199:errorcluster, "Parsed Data"=w198:variant)  [unwired: 7 in]
      n22 = Variant To Data(error in=w199, type=w196, Variant=w198) -> (data=w195:T36, error out=w197:errorcluster)
      n23 = Unbundle By Name(w195) -> ("Name"=w193:string, "Description"=w192:string, "DID Outputs"=w191:T37, "DID Inputs"=w190:T37, "PID Outputs"=w189:T37, "PID Inputs"=w188:T37, "DPIDs"=w187:T29, "DTC.Description"=w186:string, "DTC.DTC descriptor"=w178:T30, "DTC.DTC Control"=w177:T38, "Commands"=w185:cluster{"Description":string}, "Status"=w184:cluster{"Description":string}, "IO Controls"=w183:T39, "Routines"=w182:T40, "Memory Outputs"=w181:T37, "Memory Inputs"=w180:T37, "Diagnostics Basic Configuraiton.CAN Interface"=w160:T31, "Diagnostics Basic Configuraiton.Baud Rate"=w175:u32, "Diagnostics Basic Configuraiton.Diagnostic Protocol"=w174:enum16{"GMLAN", "KWP-2000", "UDS"}, "Diagnostics Basic Configuraiton.Transport Protocol"=w173:T32, "Diagnostics Basic Configuraiton.Transmit ID"=w172:u32, "Diagnostics Basic Configuraiton.Receive ID"=w171:u32, "Diagnostics Basic Configuraiton.Transmit Extension"=w170:u8, "Diagnostics Basic Configuraiton.Receive Extension"=w169:u8, "Diagnostics Basic Configuraiton.Receive UUDT ID"=w168:u32, "Diagnostics Basic Configuraiton.Enable Stream"=w167:bool, "Diagnostics Basic Configuraiton.VW TP Channel ID"=w166:u32, "Diagnostics Basic Configuraiton.Security"=w165:T41, "Diagnostics Basic Configuraiton.Fill Frame"=w164:bool, "Diagnostics Basic Configuraiton.Fill Byte"=w163:u8, "Diagnostics Basic Configuraiton.Termination"=w162:bool, "NI 986x Support.Enable"=w157:bool, "NI 986x Support.RIO Device"=w156:u16, "NI 986x Support.Bitfile"=w154:path)
      n24 = Format Into String(format string="CAN%d", w160) -> (resulting string=w159:string)  [unwired: 2 in, 1 out]
      n25 = Format Into String(format string="RIO%d", w156) -> (resulting string=w155:string)  [unwired: 2 in, 1 out]
      n26 = Bundle By Name(cluster=T1 {"Name"="", "Description"="", "Diagnostics Basic Configuraiton"={"CAN Interface"="", "Baud Rate"=0, "Diagnostic Protocol"=enum."GMLAN", "Transport Protocol"=enum."ISO TP - Normal Mode", "Transmit ID"=0, "Receive ID"=0, "Transmit Extension"=0, "Receive Extension"=0, "Receive UUDT ID"=0, "Enable Stream"=TRUE, "VW TP Channel ID"=0, "Security"={"Source DLL Path"=path "", "Security Level"=1, "Target DLL Path"=path ""}, "Fill Frame"=FALSE, "Fill Byte"=255, "Termination"=FALSE}, "DID Outputs"={"Description"="", "Frames"=[]}, "DID Inputs"={"Description"="", "Frames"=[]}, "PID Outputs"={"Description"="", "Frames"=[]}, "PID Inputs"={"Description"="", "Frames"=[]}, "DPIDs"={"Description"="", "DPIDs"=[]}, "DTC"={"Description"="", "DTC descriptor"={"DTC Byte Length"=2, "Status Byte Length"=1, "Add Data Byte Length"=1, "Byte Order"=enum."Motorola"}, "DTC Control"={"Description"="", "Signals"=[]}, "Created DTCs"=0}, "NI 986x Support"={"Enable"=FALSE, "RIO Device"="", "Bitfile"=path ""}, "Commands"={"Description"=""}, "Status"={"Description"=""}, "IO Controls"={"Description"="", "IO Control Array"=[]}, "Routines"={"Description"="", "Routine Array"=[]}, "Memory Outputs"={"Description"="", "Frames"=[]}, "Memory Inputs"={"Description"="", "Frames"=[]}, "User Defined"={"Description"="", "Groups"=[]}} ("Configuration"), "DTC.Created DTCs"=u32 10, "Name"=w193, "Description"=w192, "DID Outputs"=w191, "DID Inputs"=w190, "PID Outputs"=w189, "PID Inputs"=w188, "DPIDs"=w187, "DTC.Description"=w186, "DTC.DTC descriptor"=w178, "DTC.DTC Control"=w177, "Commands"=w185, "Status"=w184, "IO Controls"=w183, "Routines"=w182, "Memory Outputs"=w181, "Memory Inputs"=w180, "Diagnostics Basic Configuraiton.CAN Interface"=w159, "Diagnostics Basic Configuraiton.Baud Rate"=w175, "Diagnostics Basic Configuraiton.Diagnostic Protocol"=w174, "Diagnostics Basic Configuraiton.Transport Protocol"=w173, "Diagnostics Basic Configuraiton.Transmit ID"=w172, "Diagnostics Basic Configuraiton.Receive ID"=w171, "Diagnostics Basic Configuraiton.Transmit Extension"=w170, "Diagnostics Basic Configuraiton.Receive Extension"=w169, "Diagnostics Basic Configuraiton.Receive UUDT ID"=w168, "Diagnostics Basic Configuraiton.Enable Stream"=w167, "Diagnostics Basic Configuraiton.VW TP Channel ID"=w166, "Diagnostics Basic Configuraiton.Security"=w165, "Diagnostics Basic Configuraiton.Fill Frame"=w164, "Diagnostics Basic Configuraiton.Fill Byte"=w163, "Diagnostics Basic Configuraiton.Termination"=w162, "NI 986x Support.Enable"=w157, "NI 986x Support.RIO Device"=w155, "NI 986x Support.Bitfile"=w154) -> (w179:T1)
    }
    frame "5.0.0" {
      w225 = T42 {"Name"="", "Description"="", "Diagnostics Basic Configuraiton"={"CAN Interface"=enum."CAN0", "Baud Rate"=0, "Diagnostic Protocol"=enum."GMLAN", "Transport Protocol"=enum."ISO TP - Normal Mode", "Transmit ID"=0, "Receive ID"=0, "Transmit Extension"=0, "Receive Extension"=0, "Receive UUDT ID"=0, "Enable Stream"=TRUE, "VW TP Channel ID"=0, "Security"={"Source DLL Path"=path "", "Security Level"=1, "Target DLL Path"=path ""}, "Fill Frame"=FALSE, "Fill Byte"=255, "Termination"=FALSE}, "DID Outputs"={"Description"="", "Frames"=[]}, "DID Inputs"={"Description"="", "Frames"=[]}, "PID Outputs"={"Description"="", "Frames"=[]}, "PID Inputs"={"Description"="", "Frames"=[]}, "DPIDs"={"Description"="", "DPIDs"=[]}, "DTC"={"Description"="", "DTC descriptor"={"DTC Byte Length"=2, "Status Byte Length"=1, "Add Data Byte Length"=1, "Byte Order"=enum."Motorola"}, "DTC Control"={"Description"="", "Signals"=[]}, "Created DTCs"=0}, "NI 986x Support"={"Enable"=FALSE, "RIO Device"=0, "Bitfile"=path ""}, "Commands"={"Description"=""}, "Status"={"Description"=""}, "IO Controls"={"Description"="", "IO Control Array"=[]}, "Routines"={"Description"="", "Routine Array"=[]}, "Memory Outputs"={"Description"="", "Frames"=[]}, "Memory Inputs"={"Description"="", "Frames"=[]}, "User Defined"={"Description"="", "Groups"=[]}}  # Configuration
      w226 = T1 {"Name"="", "Description"="", "Diagnostics Basic Configuraiton"={"CAN Interface"="", "Baud Rate"=0, "Diagnostic Protocol"=enum."GMLAN", "Transport Protocol"=enum."ISO TP - Normal Mode", "Transmit ID"=0, "Receive ID"=0, "Transmit Extension"=0, "Receive Extension"=0, "Receive UUDT ID"=0, "Enable Stream"=TRUE, "VW TP Channel ID"=0, "Security"={"Source DLL Path"=path "", "Security Level"=1, "Target DLL Path"=path ""}, "Fill Frame"=FALSE, "Fill Byte"=255, "Termination"=FALSE}, "DID Outputs"={"Description"="", "Frames"=[]}, "DID Inputs"={"Description"="", "Frames"=[]}, "PID Outputs"={"Description"="", "Frames"=[]}, "PID Inputs"={"Description"="", "Frames"=[]}, "DPIDs"={"Description"="", "DPIDs"=[]}, "DTC"={"Description"="", "DTC descriptor"={"DTC Byte Length"=2, "Status Byte Length"=1, "Add Data Byte Length"=1, "Byte Order"=enum."Motorola"}, "DTC Control"={"Description"="", "Signals"=[]}, "Created DTCs"=0}, "NI 986x Support"={"Enable"=FALSE, "RIO Device"="", "Bitfile"=path ""}, "Commands"={"Description"=""}, "Status"={"Description"=""}, "IO Controls"={"Description"="", "IO Control Array"=[]}, "Routines"={"Description"="", "Routine Array"=[]}, "Memory Outputs"={"Description"="", "Frames"=[]}, "Memory Inputs"={"Description"="", "Frames"=[]}, "User Defined"={"Description"="", "Groups"=[]}}  # Configuration
      n27 = call-poly <vilib>:"Poly Parse.vi"("error in"=w231, "TypeDesc"=w225, "XML String In"=w232) -> ("error out"=w230:errorcluster, "Parsed Data"=w229:variant)  [unwired: 7 in]
      n28 = Variant To Data(error in=w230, type=w225, Variant=w229) -> (data=w227:T42, error out=w228:errorcluster)
      n29 = Unbundle By Name(w227) -> ("Diagnostics Basic Configuraiton.CAN Interface"=w221:T31, "Diagnostics Basic Configuraiton.Baud Rate"=w219:u32, "Diagnostics Basic Configuraiton.Diagnostic Protocol"=w218:T4, "Diagnostics Basic Configuraiton.Transport Protocol"=w217:T5, "Diagnostics Basic Configuraiton.Transmit ID"=w216:u32, "Diagnostics Basic Configuraiton.Receive ID"=w215:u32, "Diagnostics Basic Configuraiton.Transmit Extension"=w214:u8, "Diagnostics Basic Configuraiton.Receive Extension"=w213:u8, "Diagnostics Basic Configuraiton.Receive UUDT ID"=w212:u32, "Diagnostics Basic Configuraiton.Enable Stream"=w211:bool, "Diagnostics Basic Configuraiton.VW TP Channel ID"=w210:u32, "Diagnostics Basic Configuraiton.Security"=w209:T6, "Diagnostics Basic Configuraiton.Fill Frame"=w208:bool, "Diagnostics Basic Configuraiton.Fill Byte"=w207:u8, "Diagnostics Basic Configuraiton.Termination"=w206:bool, "NI 986x Support.Enable"=w205:bool, "NI 986x Support.RIO Device"=w204:u16, "NI 986x Support.Bitfile"=w202:path)
      n30 = Format Into String(format string="CAN%d", w221) -> (resulting string=w220:string)  [unwired: 2 in, 1 out]
      n31 = Format Into String(format string="RIO%d", w204) -> (resulting string=w203:string)  [unwired: 2 in, 1 out]
      n32 = Bundle By Name(cluster=w226, "Diagnostics Basic Configuraiton.CAN Interface"=w220, "Diagnostics Basic Configuraiton.Baud Rate"=w219, "Diagnostics Basic Configuraiton.Diagnostic Protocol"=w218, "Diagnostics Basic Configuraiton.Transport Protocol"=w217, "Diagnostics Basic Configuraiton.Transmit ID"=w216, "Diagnostics Basic Configuraiton.Receive ID"=w215, "Diagnostics Basic Configuraiton.Transmit Extension"=w214, "Diagnostics Basic Configuraiton.Receive Extension"=w213, "Diagnostics Basic Configuraiton.Receive UUDT ID"=w212, "Diagnostics Basic Configuraiton.Enable Stream"=w211, "Diagnostics Basic Configuraiton.VW TP Channel ID"=w210, "Diagnostics Basic Configuraiton.Security"=w209, "Diagnostics Basic Configuraiton.Fill Frame"=w208, "Diagnostics Basic Configuraiton.Fill Byte"=w207, "Diagnostics Basic Configuraiton.Termination"=w206, "NI 986x Support.Enable"=w205, "NI 986x Support.RIO Device"=w203, "NI 986x Support.Bitfile"=w202) -> (w224:T1)
    }
  }
  "Configuration" <- w10
  "error out" <- w9
